vi "Config UI.vi"(8 "error in":errorcluster) -> (0 "error out":errorcluster)   [LabVIEW 2020, in "Panther Dashboard.lvlib"]
uses:
  Panther Dashboard.lvlib
panel:
  in  "Script Request and wait for Reply Payload as a Cluster":bool caption="Checkbox"
  in  "Include vi.lib into the search for Right Click menu \"Find DQMH Broadcast Event Frames\"":bool caption="Checkbox"
  in  "Skip DQMH Framework UIs":bool caption="Checkbox"
  # "Panther Dashboard Configuration:"
  # "If this checkbox is enabled, Panther Dashboard will\nskip the DQMH Framework Default UIs and will call directly to the Scripter \nusing the current project context.\n\nThese are the DQMH Framework scripting tools where this functionality is currently implemented:\n\n* Validate DQMH Module"
  # "DQMH Framework Configuration"
  # "This right-click plugin excludes VIs in the vi.lib, user.lib, and instr.lib folders by default from the search. To restore the original behavior and include those folders in the search, add the following INI token to your LabVIEW INI file: DQMH.FindBroadcastExcludeFolders=\"\"."
  # "This applies to scripting a request and waiting for a reply. If checked, the script will include all reply indicators within a single Payload Cluster; if unchecked, it will output each payload item to a separate terminal"
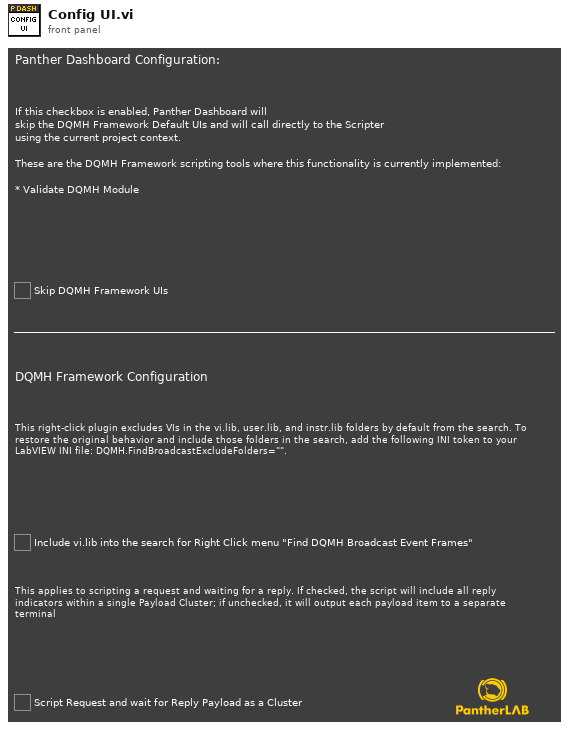
[diagram p1: front panel]
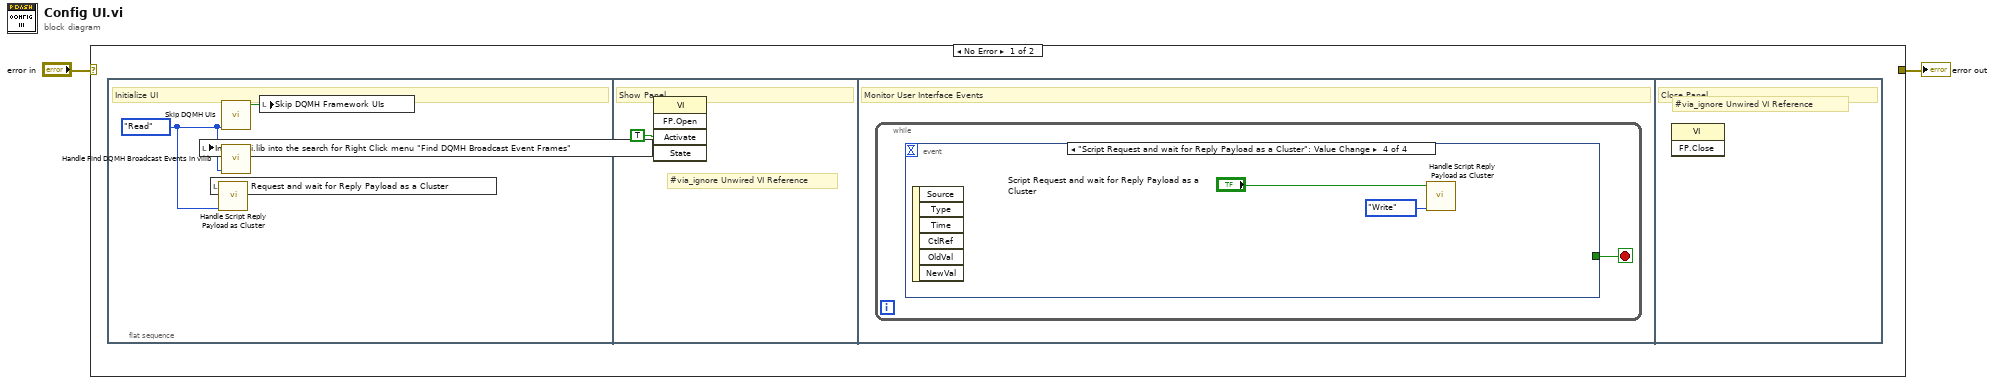
[diagram p0: block diagram]
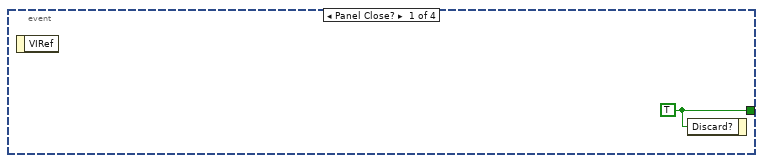
[diagram p2: hidden frame]
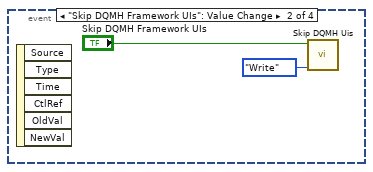
[diagram p3: hidden frame]
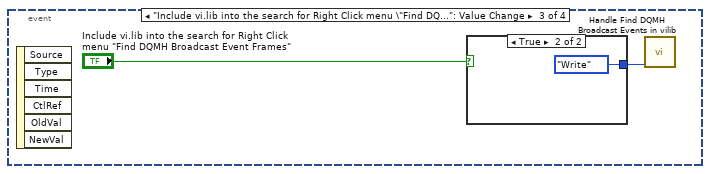
[diagram p4: hidden frame]
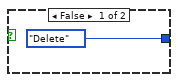
[diagram p5: hidden frame]
diagram:
  n1 = case shown="No Error" "error in" {
    selector: "error in" -> [_ w18]
    tunnel: [_ w18] -> w1
    frame No Error {
      n2 = flat-sequence {
        frame #0 {
          w4 = enum16{"Read", "Write", "Delete"}."Read" ("Action")
          # "Initialize UI"
          n3 = call "Handle Script Reply Payload as Cluster.vi"("Action"=w4) -> ("Script Payload as Cluster"=w3:bool)  [unwired: 10 in]
          n4 = local write "Script Request and wait for Reply Payload as a Cluster"(w3) -> ()
          n5 = call "Skip DQMH Uis.vi"("Action"=w4) -> ("Skip DQMH UIs"=w6:bool)  [unwired: 10 in]
          n6 = call "Handle Find DQMH Broadcast Events in vilib.vi"("Action"=w4) -> ("Exist"=w5:bool)  [unwired: 10 in]
          n7 = local write "Include vi.lib into the search for Right Click menu \"Find DQMH Broadcast Event Frames\""(w5) -> ()
          n8 = local write "Skip DQMH Framework UIs"(w6) -> ()
        }
        frame #1 {
          # "#via_ignore Unwired VI Reference"
          # "Show Panel"
          n9 = invoke class="VI" method="FP.Open"("Activate"=TRUE ("Activate?")) -> ()  [unwired: 4 in, 5 out]
        }
        frame #2 {
          # "Monitor User Interface Events"
          n10 = while {
            stop <- w8 stop-if-true
            n11 = event shown="[3] \"Script Request and wait for Reply Payload as a Cluster\": Value Change" {
              selector: _ -> [_ _ _ _]
              dyn-events: _ -> [_ _ _ _]
              timeout: _ -> [_ _ _ _]
              tunnel: [w9 _ _ _] -> w8
              event Panel Close? {
                w9 = TRUE ("Discard?")
                n12 = event-data() -> ()  [unwired: 1 in, 1 out]
                n13 = event-data("Discard?"=w9) -> ()  [unwired: 1 in, 1 out]
              }
              event "Skip DQMH Framework UIs": Value Change {
                n14 = event-data() -> ()  [unwired: 1 in, 6 out]
                n15 = call "Skip DQMH Uis.vi"("Action"=enum16{"Read", "Write", "Delete"}."Write", "Skip DQMH UIs"="Skip DQMH Framework UIs") -> ()  [unwired: 9 in, 1 out]
              }
              event "Include vi.lib into the search for Right Click menu \"Find DQMH Broadcast Event Frames\"": Value Change {
                n16 = event-data() -> ()  [unwired: 1 in, 6 out]
                n17 = case shown="True" "Include vi.lib into the search for Right Click menu \"Find DQMH Broadcast Event Frames\"" {
                  tunnel: [enum16{"Read", "Write", "Delete"}."Delete" ("Action") enum16{"Read", "Write", "Delete"}."Write" ("Action")] -> w12
                  frame False {
                  }
                  frame True {
                  }
                }
                n18 = call "Handle Find DQMH Broadcast Events in vilib.vi"("Action"=w12) -> ()  [unwired: 10 in, 1 out]
              }
              event "Script Request and wait for Reply Payload as a Cluster": Value Change {
                n19 = event-data() -> ()  [unwired: 1 in, 6 out]
                n20 = call "Handle Script Reply Payload as Cluster.vi"("Action"=enum16{"Read", "Write", "Delete"}."Write", "Script Payload as Cluster in"="Script Request and wait for Reply Payload as a Cluster") -> ()  [unwired: 9 in, 1 out]
              }
            }
          }
        }
        frame #3 {
          # "#via_ignore Unwired VI Reference"
          # "Close Panel"
          n21 = invoke class="VI" method="FP.Close"() -> ()  [unwired: 3 in, 3 out]
        }
      }
    }
    frame Error {
    }
  }
  "error out" <- w1
